vi "Functional Imaging-Remove all but one POI.vi"(8 "error in (no error)":errorcluster) -> (0 "error out":errorcluster, 1 "[POI#]":T1 {"ROI number" min=1 format="ROI %.0f"})   [LabVIEW 2020]
uses:
  Typedefs/ROI selector array-ROI vis.ctl
  xcontrol/Interface VIs/Interface typedefs/Interface-ROI selection cluster.ctl
  Typedefs/ROI ID Enum.ctl
  Global variables/gl_Functional Imaging-Global variables.vi
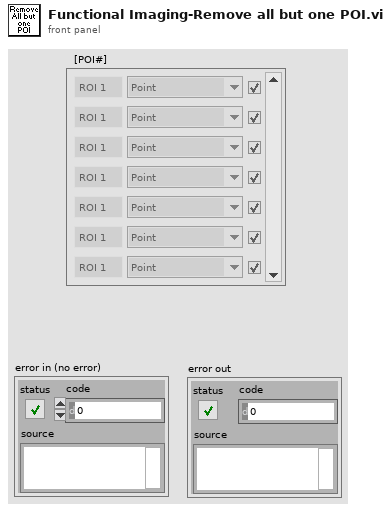
[diagram p1: front panel]
types:
  T1 = typedef "ROI selector array-ROI vis.ctl" = T2[]
  T2 = typedef "Interface-ROI selection cluster.ctl" = cluster{"ROI number":i32, "ROI ID":T3, "Visibility":bool}
  T3 = typedef "ROI ID Enum.ctl" = enum16{"Point", "MiniScan", "Comp. MiniScan", "Rectangle", "Comp. volume", "Arb. plane point", "None"}
  T4 = typedef "Functional Imging UI Refs.ctl" = cluster{"Menu ref":refnum<k9>, "Image control":refnum<vi>, "VI ref":refnum<vi>, "XGrapher":refnum<vi>, "Smoothing":refnum<vi>, "POI Averaging":refnum<vi>, "Normalize":refnum<vi>, "POI data points in each trial":refnum<vi>, "Channel":refnum<vi>, "Experiment data folder path":refnum<vi>, "[ROI vis]":refnum<vi>, "[Groups] visbl":T5, "Group Name":refnum<vi>, "POI index":refnum<vi>, "Trial No.":refnum<vi>, "Intensity Zoom":refnum<vi>, "Trial Cursor Enabled":refnum<vi>, "Number of Trials (ind 1)":refnum<vi>, "Number of Trials (ind 2)":refnum<vi>, "MiniScans Available":refnum<vi>, "POI Available":refnum<vi>, "Defer graph updates":refnum<vi>, "Waveform selector":refnum<vi>, "#of selected POI":refnum<vi>, "#of selected MiniScans":refnum<vi>, "#of selected groups":refnum<vi>, "Max Z-Projection":refnum<vi>, "Z-Plane Selector":refnum<vi>, "Index of miniscan point to visualise":refnum<vi>, "ROI vis. mode":refnum<vi>, "Total # of points":refnum<vi>, "Index of group clicked on":refnum<vi>, "Pane 1":refnum<vi>, "Pane 2":refnum<vi>, "Pane 3":refnum<vi>, "Pane 4":refnum<vi>, "Pane 5":refnum<vi>, "Pane 6":refnum<vi>, "Deselect all ROI":refnum<vi>, "Deselect all groups":refnum<vi>}
  T5 = typedef "Groups array referecne.ctl" = refnum<vi>
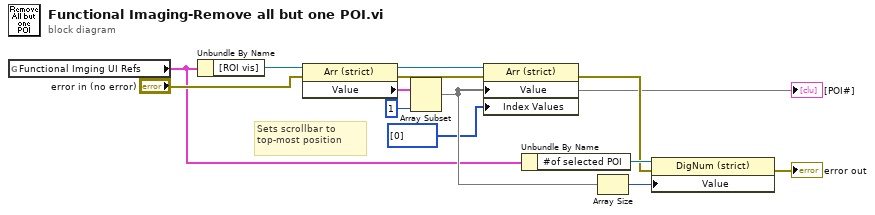
[diagram p0: block diagram]
diagram:
  # "Sets scrollbar to top-most position"
  n1 = global read "gl_Functional Imaging-Global variables.vi" "Functional Imging UI Refs"() -> (w1:T4)
  n2 = Unbundle By Name(w1) -> ("[ROI vis]"=w10:refnum<vi>)
  n3 = property on="Property Node" class="Arr (strict)"(reference=w10, error in="error in (no error)") -> (reference out=w12:refnum<vi>, error out=w8:errorcluster, "Value"=w11:T1)
  n4 = Array Subset(array=w11, length=1) -> (w4:T1)  [unwired: 1 in]
  "[POI#]" <- w4
  n5 = property on="Property Node" class="Arr (strict)"(reference=w12, error in=w8, "Value"=w4, "Index Values"=u32[] [0]) -> (error out=w5:errorcluster)  [unwired: 1 out]
  n6 = Unbundle By Name(w1) -> ("#of selected POI"=w7:refnum<vi>)
  n7 = Array Size(array=w4) -> (size(s)=w6:i32)
  n8 = property on="Property Node" class="DigNum (strict)"(reference=w7, error in=w5, "Value"=w6) -> (error out=→"error out":errorcluster)  [unwired: 1 out]
